vi "ModelParameters.GetModelParameterValue.vi"(9 "Channel Name":string, 10 "Target Name":string, 11 "GatewayIP":string) -> (0 "error out":errorcluster, 3 "Parameter Value":dbl)   [LabVIEW 2013, in "MiscHelperVIs.lvlib"]
uses:
  MiscHelperVIs.lvlib
  <vilib>/NI Veristand/Execution/ModelManager/NI VeriStand - Get Single Parameter Value.vi
  <vilib>/NI Veristand/Execution/ModelManager/NI_VS ModelManager ExecutionAPI.lvlib
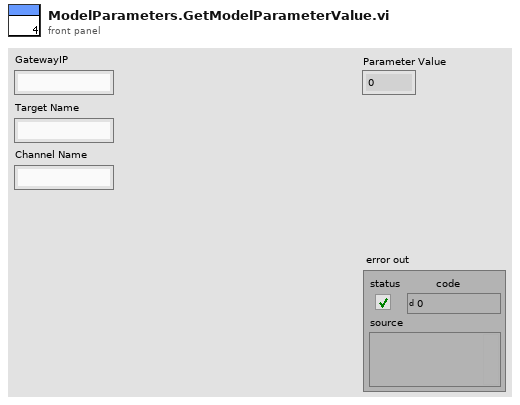
[diagram p1: front panel]
types:
  T1 = typedef "NI_VS ModelManager ExecutionAPI.lvlib/ModelManagerAPI.ctl" = refnum<k24>
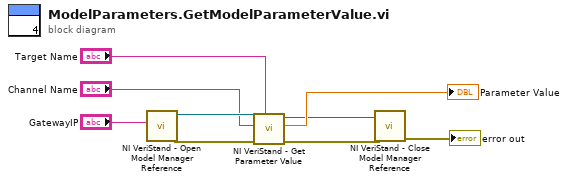
[diagram p0: block diagram]
diagram:
  n1 = call <vilib>:"NI VeriStand - Open Model Manager Reference.vi"("Gateway IP Address (\"\": localhost)"="GatewayIP") -> ("error out"=w8:errorcluster, "ModelManager"=w7:T1)  [unwired: 9 in]
  n2 = call-poly <vilib>:"NI VeriStand - Get Parameter Value.vi"("Target"="Target Name", "error in (no error)"=w8, "Parameter"="Channel Name", "ModelManager in"=w7) -> ("error out"=w2:errorcluster, "Value"=→"Parameter Value":dbl, "ModelManager out"=w1:T1)  [unwired: 5 in]
  n3 = call <vilib>:"NI VeriStand - Close Model Manager Reference.vi"("error in (no error)"=w2, "ModelManager"=w1) -> ("error out"=→"error out":errorcluster)  [unwired: 9 in]
